vi "Receive.vi"(8 "error in (no error)":errorcluster, 11 "EPU452 in":refnum<class "EPU452.lvclass">) -> (0 "error out":errorcluster, 2 "Response":string, 3 "EPU452 out":refnum<class "EPU452.lvclass">)   [LabVIEW 2018, in "EPU452.lvclass"]
uses:
  EPU452.lvclass
  EPU452.lvclass/EPU452.ctl
  <vilib>/Utility/error.llb/Clear Errors.vi
  <vilib>/Utility/error.llb/Error Cluster From Error Code.vi
panel:
  out "bap":u32
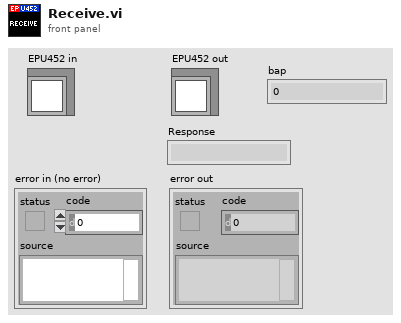
[diagram p1: front panel]
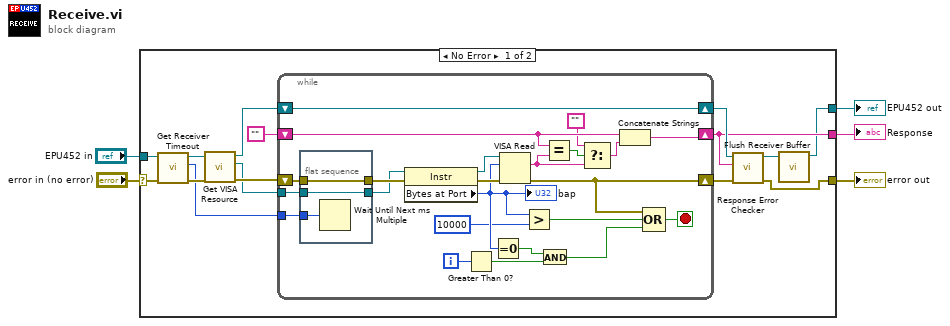
[diagram p0: block diagram]
diagram:
  n1 = case shown="No Error" "error in (no error)" {
    selector: "error in (no error)" -> [w18 w48]
    tunnel: [w6 w48] -> w4
    tunnel: [w7 w47] -> w2
    tunnel: "EPU452 in" -> [w17 w47]
    tunnel: [w9 _] -> w1
    frame No Error {
      n2 = call "Get Receiver Timeout.vi"("error in (no error)"=w18, "EPU452 in"=w17) -> ("error out"=w15:errorcluster, "Receiver Timeout"=w10:u32, "EPU452 out"=w16:refnum<class "EPU452.lvclass">)  [unwired: 7 in]
      n3 = call "Get VISA Resource.vi"("error in (no error)"=w15, "EPU452 in"=w16) -> ("error out"=w14:errorcluster, "VISA Resource"=w12:refnum<visa-resource-name>, "EPU452 out"=w13:refnum<class "EPU452.lvclass">)  [unwired: 7 in]
      n4 = while {
        shift-right: [w39] -> w9
        shift-left: "" -> [w31]
        shift-right: [w26] -> w20
        shift-left: w14 -> [w35]
        tunnel: w12 -> [w34]
        shift-right: [w37] -> w11
        shift-left: w13 -> [w37]
        tunnel: w10 -> [w27]
        i -> [w43]
        stop <- w21 stop-if-true
        n5 = flat-sequence {
          tunnel: [w46] -> w36
          tunnel: w35 -> [w46]
          tunnel: [w45] -> w33
          tunnel: w34 -> [w45]
          tunnel: w27 -> [w44]
          frame #0 {
            n6 = Wait Until Next ms Multiple(millisecond multiple=w44) -> ()  [unwired: 1 out]
          }
        }
        n7 = property class="Instr"(reference=w33, error in=w36) -> (reference out=w38:refnum<visa-resource-name>, error out=w40:errorcluster, "Bytes at Port"=w25:u32)
        "bap" <- w25
        n8 = Greater Than 0?(x=w43) -> (x > 0?=w41:bool)
        n9 = Equal To 0?(x=w25) -> (x = 0?=w42:bool)
        n10 = VISA Read(VISA resource name=w38, byte count=w25, error in (no error)=w40) -> (read buffer=w30:string, error out=w26:errorcluster)  [unwired: 2 out]
        n11 = Greater?(x=w25, y=u32 10000) -> (0:w23:bool)
        n12 = And(x=w42, y=w41) -> (x .and. y?=w22:bool)
        n13 = Equal?(x=w31, y=w30) -> (x = y?=w32:bool)
        n14 = Select(t="", s=w32, f=w30) -> (s? t:f=w29:string)
        n15 = Concatenate Strings(w31, w29) -> (w39:string)
        n16 = Compound Arithmetic op=OR(w26, w23, w22) -> (w21:bool)
      }
      n17 = call "Response Error Checker.vi"("error in (no error)"=w20, "Response in"=w9, "EPU452 in"=w11) -> ("error out"=w6:errorcluster, "EPU452 out"=w8:refnum<class "EPU452.lvclass">)  [unwired: 6 in, 1 out]
      n18 = call "Flush Receiver Buffer.vi"("EPU452 in"=w8) -> ("EPU452 out"=w7:refnum<class "EPU452.lvclass">)  [unwired: 9 in, 1 out]
    }
    frame Error {
    }
  }
  "error out" <- w4
  "EPU452 out" <- w2
  "Response" <- w1
